vi "poziomy.vi"(6 "error in (no error)":errorcluster, 7 "Wybór komory":T1, 8 "Akcja":T8=enum."Reset ramienia", 9 "LINX Resource in":T2) -> (0 "error out":errorcluster, 1 "KONIEC":bool, 2 "Aktualny stan":T9, 3 "LINX Resource out":T2)   [LabVIEW 2014]
uses:
  poziomyVIs/ParametryRuchuPoziomego.ctl
  Faza_ruchu.ctl
  poziomyVIs/RuchPoziomy.ctl
  AkcjaGFV.ctl
  parametryKomorVIs/WyborKomory.ctl
  <vilib>/MakerHub/LINX/Private/Type Defs/LINX Ref.ctl
  <vilib>/MakerHub/LINX/LMH-LINX.lvlib
  <vilib>/MakerHub/LINX/Private/Type Defs/Platform.ctl
  <vilib>/MakerHub/LINX/Private/Type Defs/Interface.ctl
  <vilib>/MakerHub/LINX/Private/Device/Type Defs/LINX Device Config.ctl
  <vilib>/MakerHub/LINX/Private/Device/Device.lvlib
  <vilib>/MakerHub/LINX/Private/Device/Type Defs/TCP Config.ctl
  <vilib>/MakerHub/LINX/Private/Device/Type Defs/Channels.ctl
  AkcjaRuchu.ctl
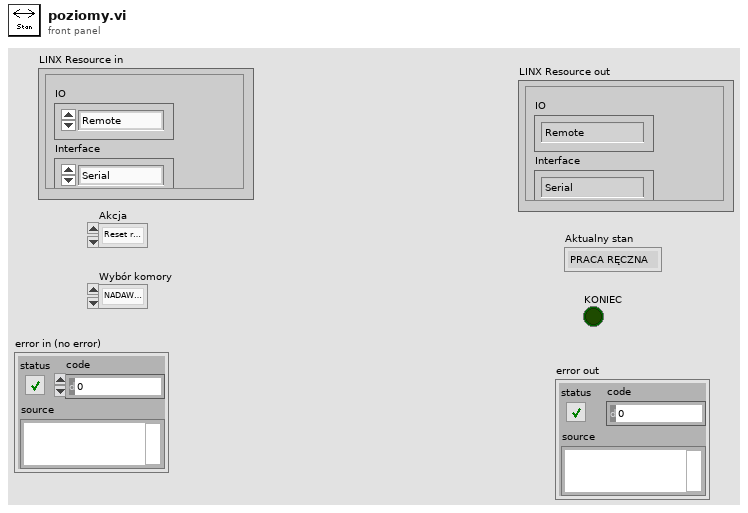
[diagram p1: front panel]
types:
  T1 = typedef "WyborKomory.ctl" = enum16{"NADAWCZA", "ODBIORCZA"}
  T2 = typedef "LMH-LINX.lvlib/LINX Ref.ctl" = cluster{"IO":T3, "Interface":T4, "LINX Device Config":T5}
  T3 = typedef "LMH-LINX.lvlib/Platform.ctl" = enum16{"Remote", "Local"}
  T4 = typedef "LMH-LINX.lvlib/Interface.ctl" = enum16{"Serial", "TCP"}
  T5 = typedef "LMH-LINX.lvlib/Device.lvlib/LINX Device Config.ctl" = cluster{"Interface":T4, "COM Port":refnum<visa-resource-name>, "TCP Configuration":T6, "Device Family":u8, "Device ID":u8, "Device Name":string, "TCP Ref":refnum<k5>, "Channels":T7}
  T6 = typedef "LMH-LINX.lvlib/Device.lvlib/TCP Config.ctl" = cluster{"IP Address":string, "Port":u16}
  T7 = typedef "LMH-LINX.lvlib/Channels.ctl" = cluster{"DI":u8[], "DO":u8[], "AI":u8[], "AO":u8[], "PWM":u8[], "QE":u8[], "UART":u8[], "I2C 2":u8[], "SPI":u8[], "CAN":u8[], "Servo":u8[], "AI Ref (V)":dbl, "AI Resolution (Bits)":u8, "AO Ref (V)":dbl, "AO Resolution (Bits)":u8}
  T8 = typedef "AkcjaRuchu.ctl" = enum16{"Init", "Reset ramienia", "Przygotuj listę", "Sprawdź", "Koniec"}
  T9 = typedef "RuchPoziomy.ctl" = enum16{"PRACA RĘCZNA", "COFAJ", "NAPRZÓD", "WYŁ."}
  T10 = typedef "Faza_ruchu.ctl" = enum16{"Ruch", "Poczekaj", "Pomiar"}
  T11 = typedef "AkcjaGFV.ctl" = enum16{"Czytaj", "Zapisz", "Reset"}
  T12 = typedef "ParametryRuchuPoziomego.ctl" = cluster{"Faza ruchu poziomego":T10, "Nr pozycji poziomej":i32, "Kolor czujnika":bool, "Lista punków w poziomie":i32[]}
  T13 = typedef "WejsciaParametry.ctl" = cluster{"LEWO":bool, "PRAWO":bool, "GÓRA":bool, "Dӣ":bool, "Stop":bool, "Start":bool, "Praca ręczna":bool, "Komora":bool, "Rodzaj pomiarów":T14}
  T14 = typedef "RodzajPomiarow.ctl" = enum16{"Izolacyjność Akustyczna"}
  T15 = typedef "PinoutLista.ctl" = cluster{"LEWO":u8, "PRAWO":u8, "GÓRA":u8, "Dӣ":u8, "CZUJNIK":u8, "I2C ADRES":u8}
  T16 = typedef "Gotowosc.ctl" = cluster{"Poziomy":bool, "Pionowy":bool}
  T17 = typedef "WyjsciaParametry.ctl" = cluster{"Nad. lewo":bool, "Nad.  prawo":bool, "Nad.  góra":bool, "Nad. dół":bool, "Działanie":bool, "Pomiar":bool, "Odb. dół":bool, "Odb.  góra":bool, "Odb.  prawo":bool, "Odb. lewo":bool, "Punkty pom. info":string}
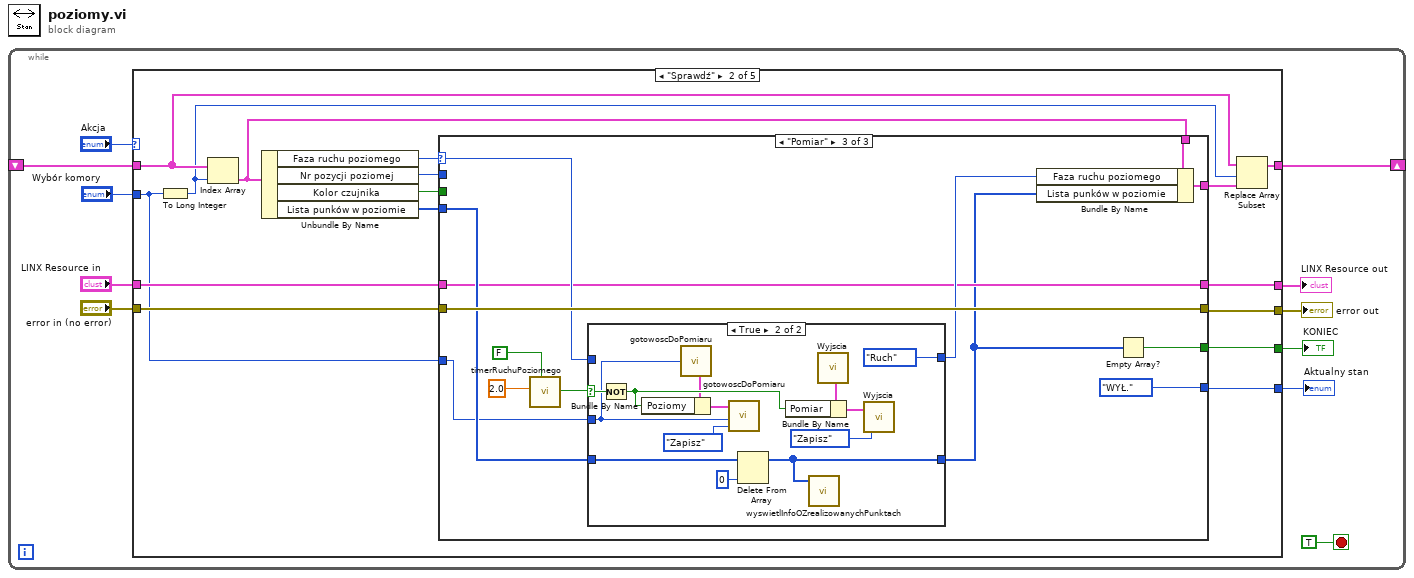
[diagram p0: block diagram]
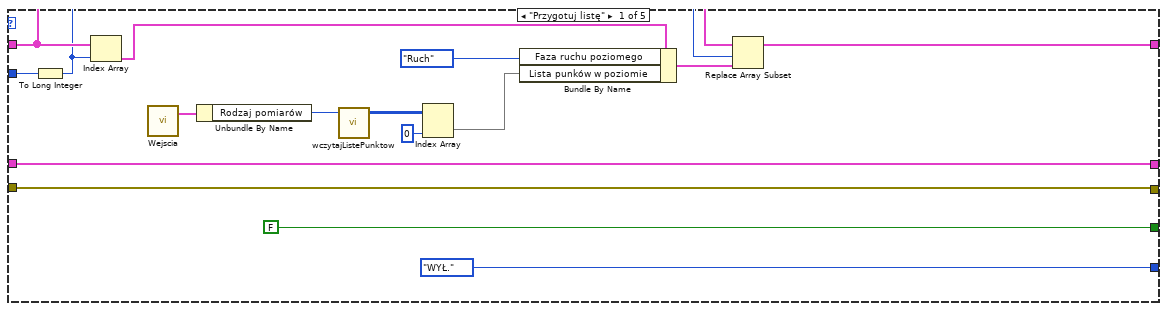
[diagram p2: hidden frame]
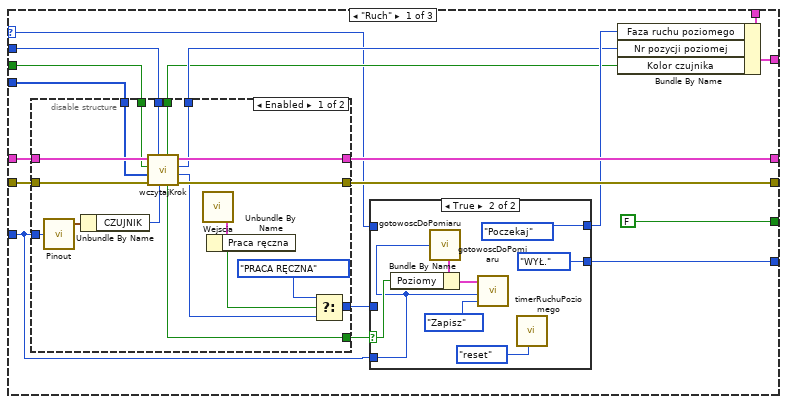
[diagram p3: hidden frame]
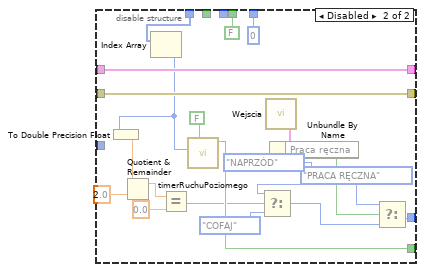
[diagram p4: hidden frame]
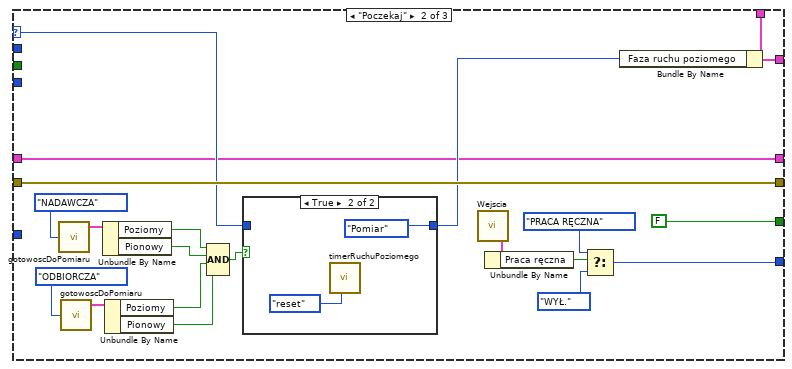
[diagram p6: hidden frame]
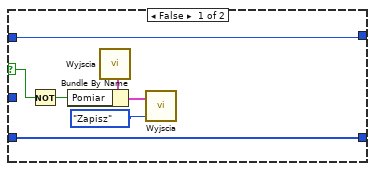
[diagram p8: hidden frame]
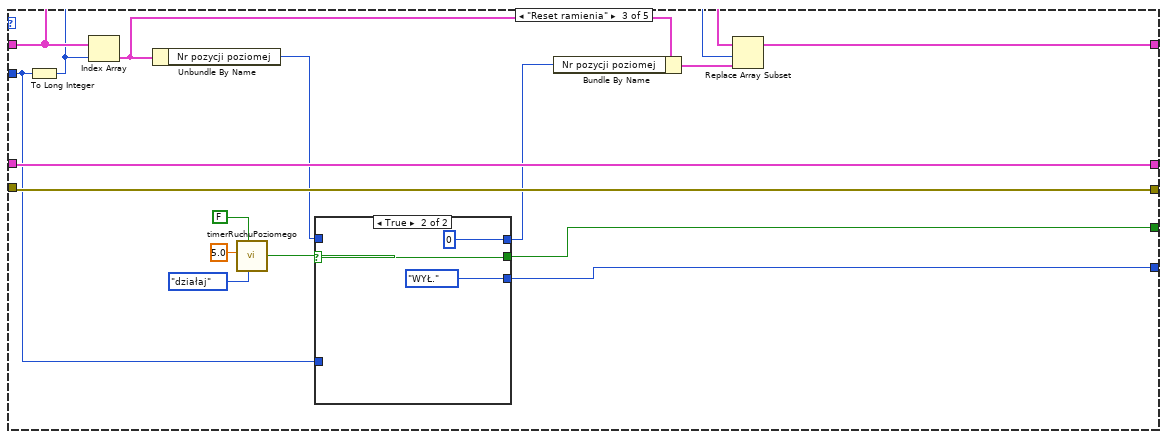
[diagram p9: hidden frame]
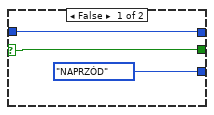
[diagram p10: hidden frame]
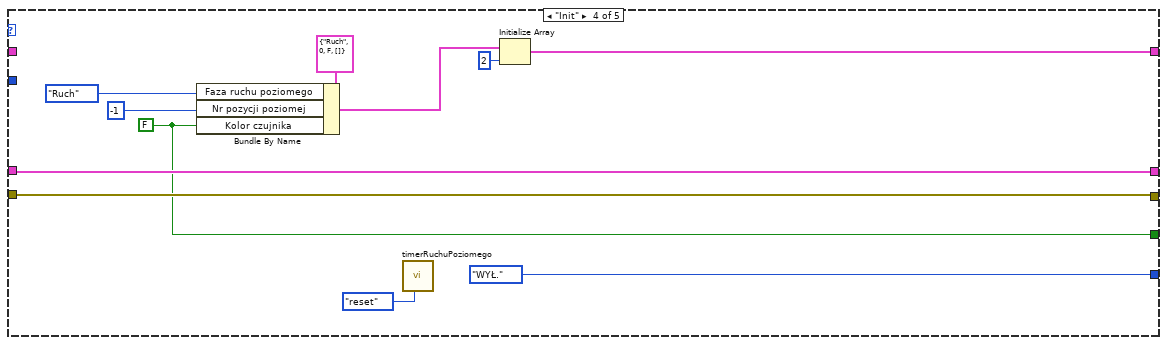
[diagram p11: hidden frame]
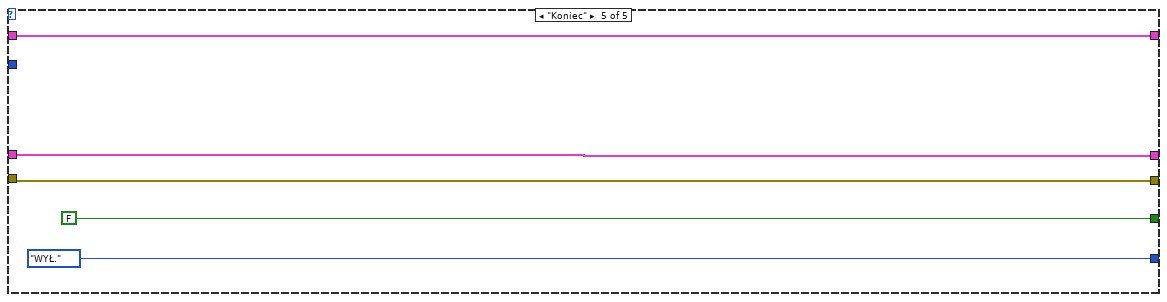
[diagram p12: hidden frame]
diagram:
  n1 = while {
    shift-right: [w3] -> _
    shift-left: _ -> [w2]
    stop <- TRUE stop-if-true
    n2 = case shown="\"Sprawdź\"" "Akcja" {
      tunnel: "LINX Resource in" -> [w27 w39 w181 w199 w205]
      tunnel: "error in (no error)" -> [w26 w43 w180 w198 w204]
      tunnel: [w27 w38 w181 w199 w205] -> w9
      tunnel: [w26 w42 w180 w198 w204] -> w7
      tunnel: [RuchPoziomy."WYŁ." ("Stan poziomy") w41 w183 RuchPoziomy."WYŁ." ("Stan poziomy") RuchPoziomy."WYŁ." ("Stan poziomy")] -> w6
      tunnel: [FALSE ("Poziomy") w40 w182 w193 FALSE ("empty?")] -> w5
      tunnel: w2 -> [w22 w33 w175 _ w201]
      tunnel: [w23 w30 w173 w190 w201] -> w3
      tunnel: "Wybór komory" -> [w17 w29 w168 _ _]
      frame "Przygotuj listę" {
        n3 = To Long Integer(number=w17) -> (32bit integer=w18:i32)
        n4 = Index Array(array=w22, index=w18) -> (element=w19:T12)
        n5 = call "Wejscia.vi"() -> ("Wyjście"=w16:T13)  [unwired: 5 in]
        n6 = Unbundle By Name(w16) -> ("Rodzaj pomiarów"=w15:T14)
        n7 = call "wczytajListePunktow.vi"(5:w15) -> ("Wspolrzedne katowe"=w14:i32[][])  [unwired: 4 in]
        n8 = Index Array(array=w14, index (col)=0 ("disabled index (col)")) -> (element=w12:i32[])  [unwired: 1 in]
        n9 = Bundle By Name(cluster=w19, "Faza ruchu poziomego"=Faza_ruchu."Ruch" ("Faza ruchu"), "Lista punków w poziomie"=w12) -> (w20:T12)
        n10 = Replace Array Subset(array=w22, new element=w20, index=w18) -> (w23:T12[])
      }
      frame "Sprawdź" {
        n11 = To Long Integer(number=w29) -> (32bit integer=w31:i32)
        n12 = Index Array(array=w33, index=w31) -> (element=w28:T12)
        n13 = Unbundle By Name(w28) -> ("Faza ruchu poziomego"=w37:T10, "Nr pozycji poziomej"=w36:i32, "Kolor czujnika"=w35:bool, "Lista punków w poziomie"=w34:i32[])
        n14 = case shown="\"Pomiar\"" w37 {
          selector: w37 -> [w44 w128 w143]
          tunnel: [w56 w120 w138] -> w38
          tunnel: w43 -> [w61 w130 w146]
          tunnel: [w60 w130 w146] -> w42
          tunnel: w35 -> [w48 _ _]
          tunnel: w36 -> [w54 _ _]
          tunnel: w34 -> [w47 _ w142]
          tunnel: [w58 w122 RuchPoziomy."WYŁ." ("Stan poziomy")] -> w41
          tunnel: [FALSE ("empty?") FALSE ("empty?") w140] -> w40
          tunnel: [w50 w119 w135] -> w32
          tunnel: w39 -> [w57 w120 w138]
          tunnel: w29 -> [w45 _ w134]
          tunnel: w28 -> [w46 w118 w136]
          frame "Ruch" {
            n15 = disable-structure shown="Enabled" {
              disable-tunnel: w61 -> [w79 w97]
              disable-tunnel: [w78 w97] -> w60
              disable-tunnel: [w74 w83] -> w59
              disable-tunnel: w57 -> [w72 w98]
              disable-tunnel: [w71 w98] -> w56
              disable-tunnel: [w70 w93] -> w55
              disable-tunnel: w54 -> [w69 _]
              disable-tunnel: [w68 0 ("Nowy nr pozycji poziomej")] -> w52
              disable-tunnel: [w67 FALSE ("Kolor na czujniku")] -> w51
              disable-tunnel: w45 -> [w64 _]
              disable-tunnel: w48 -> [w63 _]
              disable-tunnel: w47 -> [w62 w95]
              frame Enabled {
                n16 = call "Pinout.vi"("Wybór komory"=w64) -> ("Wyjście"=w66:T15)  [unwired: 4 in]
                n17 = Unbundle By Name(w66) -> ("CZUJNIK"=w65:u8)
                n18 = call "wczytajKrok.vi"("CZUJNIK"=w65, "Nr pozycji poziomej"=w69, "error in (no error)"=w79, "Lista punków w poziomie"=w62, "Kolor czujnika"=w63, "LINX Resource in"=w72) -> ("error out"=w78:errorcluster, "Faza ruchu wstępna"=w73:T9, "Nowy nr pozycji poziomej"=w68:i32, "LINX Resource"=w71:T2, "Czy na żądanej pozycji?"=w70:bool, "Kolor na czujniku"=w67:bool)
                n19 = call "Wejscia.vi"() -> ("Wyjście"=w75:T13)  [unwired: 5 in]
                n20 = Unbundle By Name(w75) -> ("Praca ręczna"=w77:bool)
                n21 = Select(t=RuchPoziomy."PRACA RĘCZNA" ("Stan pracy ręcznej - poz"), s=w77, f=w73) -> (s? t:f=w74:T9)
              }
              frame Disabled {
                n22 = Index Array(array=w95) -> (element=w81:i32)  [unwired: 1 in]
                n23 = To Double Precision Float(number=w81) -> (double precision float=w80:dbl)
                n24 = Quotient & Remainder(x=w80, y=2.0) -> (x-y*floor(x/y)=w82:dbl)  [unwired: 1 out]
                n25 = Equal?(x=w82, y=0.0) -> (x = y?=w90:bool)
                n26 = call "timerRuchuPoziomego.vi"("pauza"=FALSE, "Czas"=w81) -> ("czy czas upłynął"=w93:bool)  [unwired: 9 in]
                n27 = Select(t=RuchPoziomy."NAPRZÓD" ("Faza ruchu wstępna"), s=w90, f=RuchPoziomy."COFAJ") -> (s? t:f=w84:T9)
                n28 = call "Wejscia.vi"() -> ("Wyjście"=w85:T13)  [unwired: 5 in]
                n29 = Unbundle By Name(w85) -> ("Praca ręczna"=w87:bool)
                n30 = Select(t=RuchPoziomy."PRACA RĘCZNA" ("Stan pracy ręcznej - poz"), s=w87, f=w84) -> (s? t:f=w83:T9)
              }
            }
            n31 = case shown="True" w55 {
              selector: w55 -> [_ w106]
              tunnel: w44 -> [w101 _]
              tunnel: [w101 Faza_ruchu."Poczekaj" ("f")] -> w53
              tunnel: w59 -> [w100 _]
              tunnel: [w100 RuchPoziomy."WYŁ." ("Stan poziomy")] -> w58
              tunnel: w45 -> [_ w102]
              frame False {
              }
              frame True {
                n32 = call "gotowoscDoPomiaru.vi"("Wybór komory"=w102) -> ("Gotowość wyjście"=w103:T16)  [unwired: 4 in]
                n33 = Bundle By Name(cluster=w103, "Poziomy"=w106) -> (w108:T16)
                n34 = call "gotowoscDoPomiaru.vi"("Akcja"=AkcjaGFV."Zapisz", "Wybór komory"=w102, "Gotowość"=w108) -> ()  [unwired: 2 in, 1 out]
                n35 = call "timerRuchuPoziomego.vi"("Czynność"=enum16{"reset", "działaj"}."reset") -> ()  [unwired: 10 in, 1 out]
              }
            }
            n36 = Bundle By Name(cluster=w46, "Faza ruchu poziomego"=w53, "Nr pozycji poziomej"=w52, "Kolor czujnika"=w51) -> (w50:T12)
          }
          frame "Poczekaj" {
            n37 = call "gotowoscDoPomiaru.vi"("Wybór komory"=WyborKomory."NADAWCZA") -> ("Gotowość wyjście"=w129:T16)  [unwired: 4 in]
            n38 = call "gotowoscDoPomiaru.vi"("Wybór komory"=WyborKomory."ODBIORCZA") -> ("Gotowość wyjście"=w117:T16)  [unwired: 4 in]
            n39 = Unbundle By Name(w129) -> ("Poziomy"=w115:bool, "Pionowy"=w114:bool)
            n40 = Unbundle By Name(w117) -> ("Poziomy"=w113:bool, "Pionowy"=w112:bool)
            n41 = Compound Arithmetic op=AND(w115, w114, w113, w112) -> (w116:bool)
            n42 = case shown="True" w116 {
              tunnel: w128 -> [w131 _]
              tunnel: [w131 Faza_ruchu."Pomiar" ("t")] -> w121
              frame False {
              }
              frame True {
                n43 = call "timerRuchuPoziomego.vi"("Czynność"=enum16{"reset", "działaj"}."reset") -> ()  [unwired: 10 in, 1 out]
              }
            }
            n44 = call "Wejscia.vi"() -> ("Wyjście"=w124:T13)  [unwired: 5 in]
            n45 = Unbundle By Name(w124) -> ("Praca ręczna"=w126:bool)
            n46 = Select(t=RuchPoziomy."PRACA RĘCZNA" ("Stan pracy ręcznej - poz"), s=w126, f=RuchPoziomy."WYŁ." ("Stan poziomy")) -> (s? t:f=w122:T9)
            n47 = Bundle By Name(cluster=w118, "Faza ruchu poziomego"=w121) -> (w119:T12)
          }
          frame "Pomiar" {
            n48 = call "timerRuchuPoziomego.vi"("pauza"=FALSE, "Czas"=2.0) -> ("czy czas upłynął"=w144:bool)  [unwired: 9 in]
            n49 = case shown="True" w144 {
              selector: w144 -> [w149 w160]
              tunnel: w143 -> [w154 _]
              tunnel: [w154 Faza_ruchu."Ruch" ("Faza ruchu")] -> w139
              tunnel: w142 -> [w153 w161]
              tunnel: [w153 w155] -> w137
              tunnel: w134 -> [_ w156]
              frame False {
                n50 = Not(x=w149) -> (.not. x?=w148:bool)
                n51 = call "Wyjscia.vi"() -> ("Wyjście"=w152:T17)  [unwired: 5 in]
                n52 = Bundle By Name(cluster=w152, "Pomiar"=w148) -> (w151:T17)
                n53 = call "Wyjscia.vi"("Akcja"=AkcjaGFV."Zapisz", "Wejście"=w151) -> ()  [unwired: 3 in, 1 out]
              }
              frame True {
                n54 = Not(x=w160) -> (.not. x?=w159:bool)
                n55 = call "gotowoscDoPomiaru.vi"("Wybór komory"=w156) -> ("Gotowość wyjście"=w157:T16)  [unwired: 4 in]
                n56 = Bundle By Name(cluster=w157, "Poziomy"=w159) -> (w166:T16)
                n57 = call "gotowoscDoPomiaru.vi"("Akcja"=AkcjaGFV."Zapisz", "Wybór komory"=w156, "Gotowość"=w166) -> ()  [unwired: 2 in, 1 out]
                n58 = Delete From Array(array=w161, index=0) -> (array with subset deleted=w155:i32[])  [unwired: 1 in, 1 out]
                n59 = call "wyswietlInfoOZrealizowanychPunktach.vi"("Lista punktow"=w155) -> ()  [unwired: 5 in]
                n60 = call "Wyjscia.vi"() -> ("Wyjście"=w164:T17)  [unwired: 5 in]
                n61 = Bundle By Name(cluster=w164, "Pomiar"=w159) -> (w163:T17)
                n62 = call "Wyjscia.vi"("Akcja"=AkcjaGFV."Zapisz", "Wejście"=w163) -> ()  [unwired: 3 in, 1 out]
              }
            }
            n63 = Bundle By Name(cluster=w136, "Faza ruchu poziomego"=w139, "Lista punków w poziomie"=w137) -> (w135:T12)
            n64 = Empty Array?(array=w137) -> (empty?=w140:bool)
          }
        }
        n65 = Replace Array Subset(array=w33, new element=w32, index=w31) -> (w30:T12[])
      }
      frame "Reset ramienia" {
        n66 = To Long Integer(number=w168) -> (32bit integer=w174:i32)
        n67 = Index Array(array=w175, index=w174) -> (element=w169:T12)
        n68 = Unbundle By Name(w169) -> ("Nr pozycji poziomej"=w172:i32)
        n69 = call "timerRuchuPoziomego.vi"("Czynność"=enum16{"reset", "działaj"}."działaj", "pauza"=FALSE, "Czas"=5.0) -> ("czy czas upłynął"=w177:bool)  [unwired: 8 in]
        n70 = case shown="True" w177 {
          selector: w177 -> [w184 w187]
          tunnel: [w185 0] -> w171
          tunnel: [RuchPoziomy."NAPRZÓD" ("Stan poziomy") RuchPoziomy."WYŁ." ("Stan poziomy")] -> w183
          tunnel: w172 -> [w185 _]
          tunnel: [w184 w187] -> w182
          tunnel: w168 -> [_ _]
          frame False {
          }
          frame True {
          }
        }
        n71 = Bundle By Name(cluster=w169, "Nr pozycji poziomej"=w171) -> (w170:T12)
        n72 = Replace Array Subset(array=w175, new element=w170, index=w174) -> (w173:T12[])
      }
      frame "Init" {
        w193 = FALSE
        n73 = Bundle By Name(cluster=T12 {"Faza ruchu poziomego"=enum."Ruch", "Nr pozycji poziomej"=0, "Kolor czujnika"=FALSE, "Lista punków w poziomie"=[]} ("Parametry ruchu poziomego"), "Faza ruchu poziomego"=Faza_ruchu."Ruch" ("Faza ruchu"), "Nr pozycji poziomej"=-1, "Kolor czujnika"=w193) -> (w192:T12)
        n74 = call "timerRuchuPoziomego.vi"("Czynność"=enum16{"reset", "działaj"}."reset") -> ()  [unwired: 10 in, 1 out]
        n75 = Initialize Array(w192, 2 ("dimension size")) -> (w190:T12[])
      }
      frame "Koniec" {
      }
    }
    "error out" <- w7
    "LINX Resource out" <- w9
    "Aktualny stan" <- w6
    "KONIEC" <- w5
  }
